vi "DS4Monitor.vi"() -> ()   [LabVIEW 2024]
uses:
  <vilib>/Utility/inputDevices.llb/joystickAcquire.vi
  <vilib>/Utility/inputDevices.llb/closeJoystick.vi
panel:
  out "D-Pad Input":T1
  out "DS4 Button Input":T2
  out "joystick info":T3(array[cluster])
  out "Right Stick":cluster{i32[], i32[]}(graph)
  out "Left Stick":cluster{i32[], i32[]}(graph)
  out "error out":errorcluster
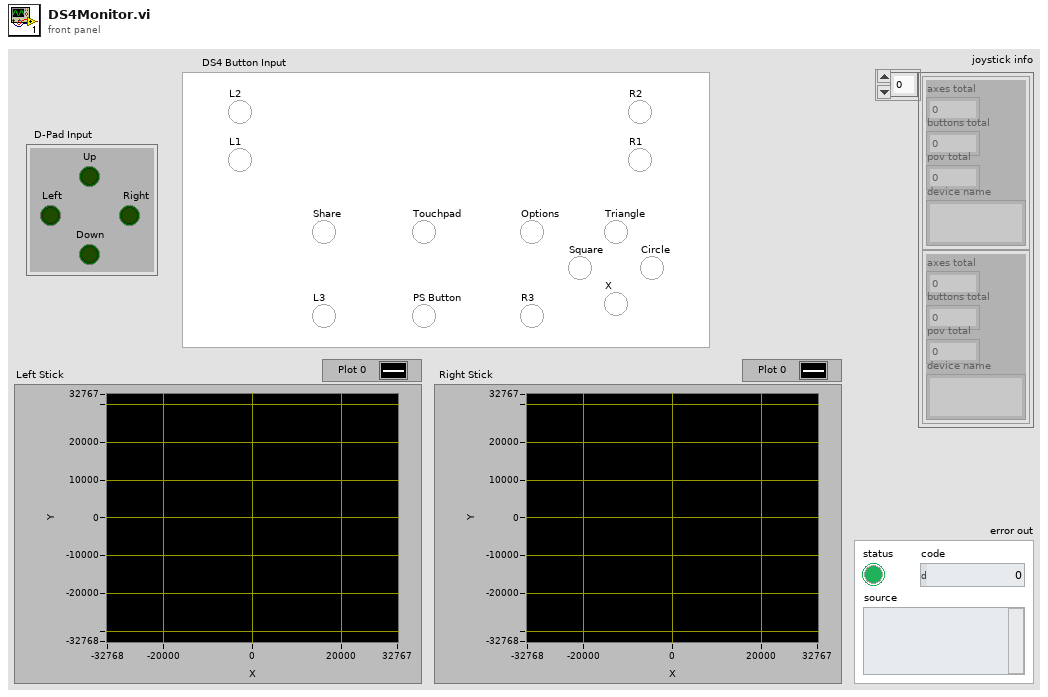
[diagram p1: front panel]
types:
  T1 = cluster{"Up":bool, "Right":bool, "Down":bool, "Left":bool}
  T2 = cluster{"X":bool, "Square":bool, "Circle":bool, "Triangle":bool, "L1":bool, "R1":bool, "L2":bool, "R2":bool, "Options":bool, "Share":bool, "L3":bool, "R3":bool, "Touchpad":bool, "PS Button":bool}
  T3 = cluster{"axes total":u32, "buttons total":u32, "pov total":u32, "device name":string}[]
  T4 = cluster{"X axis":i32, "Y axis":i32, "Z axis":i32, "X axis rotation":i32, "Y axis rotation":i32, "Z axis rotation":i32, "U axis":i32, "V axis":i32}
  T5 = cluster{"button 1":bool, "button 2":bool, "button 3":bool, "button 4":bool, "button 5":bool, "button 6":bool, "button 7":bool, "button 8":bool, "button 9":bool, "button 10":bool, "button 11":bool, "button 12":bool, "button 13":bool, "button 14":bool, "button 15":bool, "button 16":bool, "button 17":bool, "button 18":bool, "button 19":bool, "button 20":bool, "button 21":bool, "button 22":bool, "button 23":bool, "button 24":bool, "button 25":bool, "button 26":bool, "button 27":bool, "button 28":bool, "button 29":bool, "button 30":bool, "button 31":bool, "button 32":bool}
  T6 = cluster{"pov 1":i32, "pov 2":i32, "pov 3":i32, "pov 4":i32}
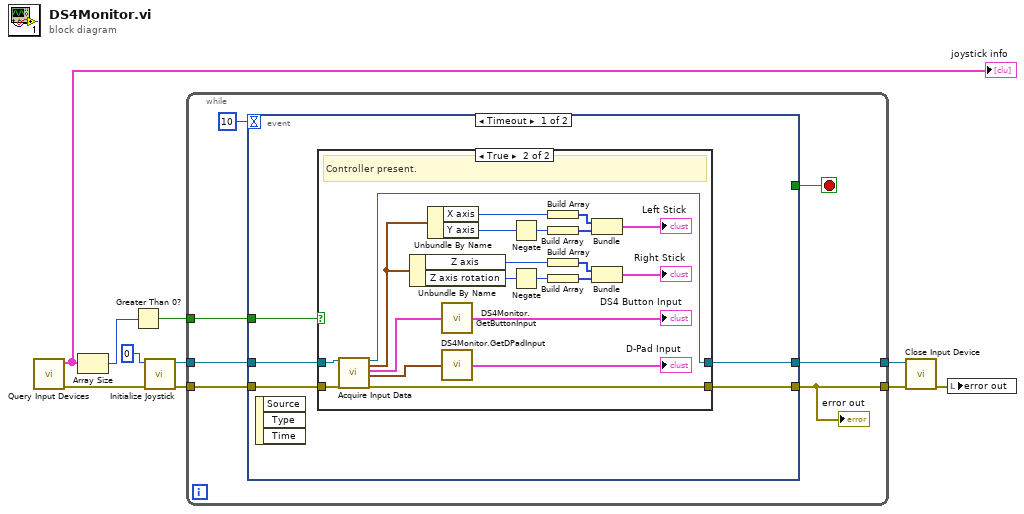
[diagram p0: block diagram]
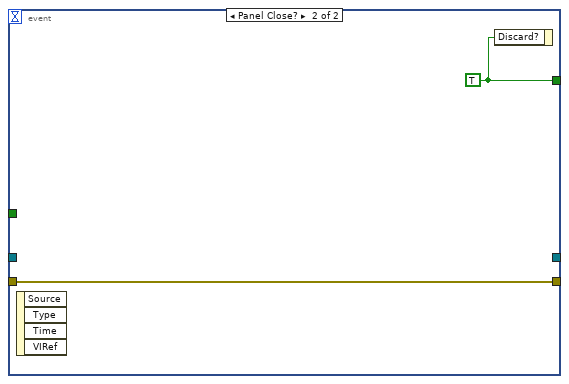
[diagram p3: hidden frame]
diagram:
  n1 = call <vilib>:"Query Input Devices.vi"() -> ("error out"=w4:errorcluster, "joystick info"=w3:T3)  [unwired: 8 in, 2 out]
  "joystick info" <- w3
  n2 = Array Size(array=w3) -> (size(s)=w2:i32)
  n3 = Greater Than 0?(x=w2) -> (x > 0?=w1:bool)
  n4 = call <vilib>:"Initialize Joystick.vi"("error in (no error)"=w4, "device index"=0) -> ("error out"=w10:errorcluster, "device ID"=w9:refnum<k1>)  [unwired: 8 in]
  n5 = while {
    tunnel: w10 -> [w16]
    tunnel: w9 -> [w17]
    tunnel: [w13] -> w8
    tunnel: [w12] -> w6
    tunnel: w1 -> [w11]
    stop <- w14 stop-if-true
    n6 = event shown="[0] Timeout" {
      selector: _ -> [_ _]
      dyn-events: _ -> [_ _]
      timeout: 10 -> [_ _]
      tunnel: w17 -> [w22 _]
      tunnel: w16 -> [w21 w46]
      tunnel: [_ w47] -> w14
      tunnel: [w20 w46] -> w13
      tunnel: [w19 _] -> w12
      tunnel: w11 -> [w18 _]
      event Timeout {
        n7 = event-data() -> ()  [unwired: 1 in, 3 out]
        n8 = case shown="True" w18 {
          tunnel: w22 -> [w23 w45]
          tunnel: w21 -> [w24 w44]
          tunnel: [w24 w27] -> w20
          tunnel: [w23 w43] -> w19
          frame False {
            # "Controller not present."
          }
          frame True {
            # "Controller present."
            n9 = call-poly <vilib>:"Acquire Input Data.vi"("device ID"=w45, "error in (no error)"=w44) -> ("device ID"=w43:refnum<k1>, "axis info"=w35:T4, "button info"=w36:T5, "direction info"=w26:T6, "error out"=w27:errorcluster)  [unwired: 13 in]
            n10 = Unbundle By Name(w35) -> ("Z axis"=w33:i32, "Z axis rotation"=w34:i32)
            n11 = Unbundle By Name(w35) -> ("X axis"=w42:i32, "Y axis"=w41:i32)
            n12 = call "DS4Monitor.GetButtonInput.vi"("button info"=w36) -> ("DS4 Button Input"=→"DS4 Button Input":T2)
            n13 = call "DS4Monitor.GetDPadInput.vi"("direction info"=w26) -> ("D-Pad Input"=→"D-Pad Input":T1)
            n14 = Negate(x=w41) -> (-x=w37:i32)
            n15 = Negate(x=w34) -> (-x=w32:i32)
            n16 = Build Array(w42) -> (w40:i32[])
            n17 = Build Array(w37) -> (w39:i32[])
            n18 = Build Array(w33) -> (w31:i32[])
            n19 = Build Array(w32) -> (w30:i32[])
            n20 = Bundle(w40, w39) -> (→"Left Stick":cluster{i32[], i32[]})  [unwired: 1 in]
            n21 = Bundle(w31, w30) -> (→"Right Stick":cluster{i32[], i32[]})  [unwired: 1 in]
          }
        }
      }
      event Panel Close? {
        w47 = TRUE
        n22 = event-data() -> ()  [unwired: 1 in, 4 out]
        n23 = event-data("Discard?"=w47) -> ()  [unwired: 1 in, 1 out]
      }
    }
    "error out" <- w13
  }
  n24 = call-poly <vilib>:"Close Input Device.vi"("error in (no error)"=w8, "device ID"=w6) -> ("error out"=w7:errorcluster)  [unwired: 8 in]
  n25 = local write "error out"(w7) -> ()
